vi "SCM1 Ramp and Soak.vi"(2 "Point #":i32, 4 "Parameters":dbl[](array[numeric]) format="%.3e", 5 "GPIB":refnum<visa-resource-name>) -> (0 "Stop":bool, 1 "Data Out":dbl[](array[numeric]) format="%.2f")   [LabVIEW 2025]
doc: "Author: Scott Hannahs <sth@magnet.fsu.edu>\n\nThis software is licensed for use under the “MIT License\"\nCopyright (c) 2025 Scott Hannahs, sth@sth@magnet.sthnet.net\n\nPermission is hereby granted, free of charge, to any person obtaining a copy of this software and associated documentation files (the \"Software\"), to deal in the Software without restriction, including without limitation the rights to use, copy, modify, merge, publish, distribute, sublicense, and/or sell copies of the Software, and to permit persons to whom the Software is furnished to do so, subject to the following conditions: The above copyright notice and this permission notice shall be included in all copies or substantial portions of the Software.\n\nTHE SOFTWARE IS PROVIDED \"AS IS\", WITHOUT WARRANTY OF ANY KIND, EXPRESS OR IMPLIED, INCLUDING BUT NOT LIMITED TO THE WARRANTIES OF MERCHANTABILITY, FITNESS FOR A PARTICULAR PURPOSE AND NONINFRINGEMENT. IN NO EVENT SHALL THE AUTHORS OR COPYRIGHT HOLDERS BE LIABLE FOR ANY CLAIM, DAMAGES OR OTHER LIABILITY, WHETHER IN AN ACTION OF CONTRACT, TORT OR OTHERWISE, ARISING FROM, OUT OF OR IN CONNECTION WITH THE SOFTWARE OR THE USE OR OTHER DEALINGS IN THE SOFTWARE."
panel:
  out "Starting Field":dbl format="%.2f"
  # "Step Size"
  # "Final Field T"
  # "Ramp Rate A/s"
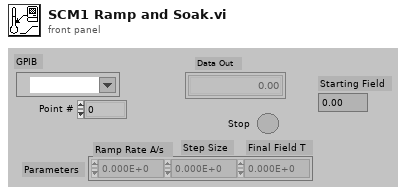
[diagram p1: front panel]
types:
  T1 = cluster{"Parameters[0]":dbl, "Parameters[1]":dbl, "Parameters[2]":dbl}
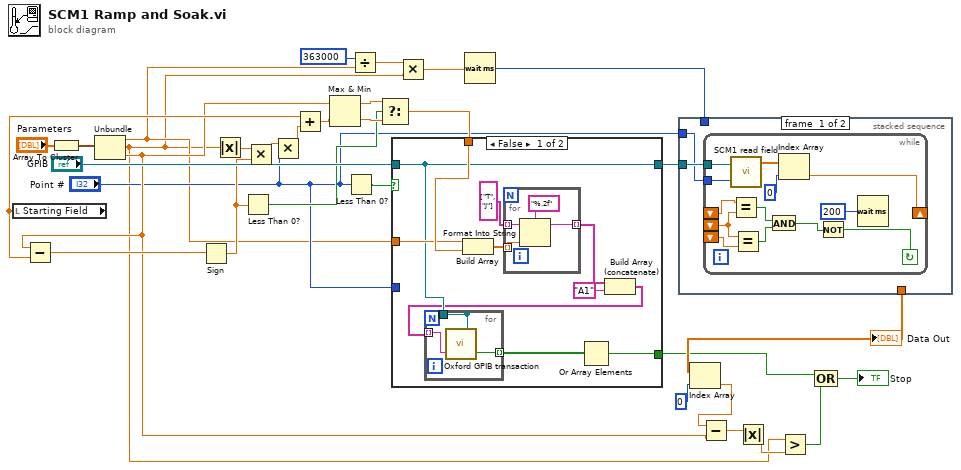
[diagram p0: block diagram]
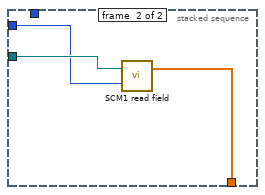
[diagram p2: hidden frame]
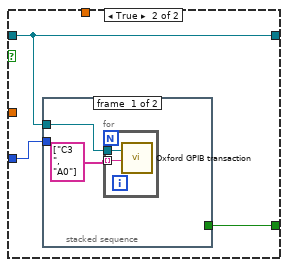
[diagram p3: hidden frame]
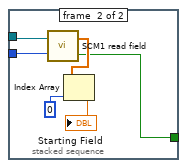
[diagram p4: hidden frame]
diagram:
  n1 = local read "Starting Field"() -> (w21:dbl)
  n2 = Array To Cluster(array="Parameters") -> (cluster=w19:T1)
  n3 = Unbundle(w19) -> ("Parameters[0]"=w6:dbl, "Parameters[1]"=w3:dbl, "Parameters[2]"=w12:dbl)
  n4 = Subtract(x=w12, y=w21) -> (x-y=w30:dbl)
  n5 = Sign(1:w30) -> (0:w23:dbl)
  n6 = Absolute Value(x=w3) -> (abs(x)=w28:dbl)
  n7 = Less Than 0?(x=w23) -> (x < 0?=w22:bool)
  n8 = Multiply(x=w28, y=w23) -> (x*y=w29:dbl)
  n9 = Multiply(x=w29, y="Point #") -> (x*y=w32:dbl)
  n10 = Add(x=w21, y=w32) -> (x+y=w27:dbl)
  n11 = Max & Min(x=w12, y=w27) -> (max(x,y)=w25:dbl, min(x,y)=w24:dbl)
  n12 = Less Than 0?(x="Point #") -> (x < 0?=w20:bool)
  n13 = Divide(x=363000, y=w6) -> (x/y=w4:dbl)
  n14 = Select(t=w25, s=w22, f=w24) -> (s? t:f=w26:dbl)
  n15 = case shown="False" w20 {
    tunnel: "GPIB" -> [w38 w52]
    tunnel: [w38 w52] -> w16
    tunnel: w26 -> [w40 _]
    tunnel: "Point #" -> [_ w51]
    tunnel: [w36 w50] -> w10
    tunnel: w6 -> [w39 _]
    frame False {
      n16 = Build Array(w39, w40) -> (w41:dbl[])
      n17 = for {
        tunnel: w41 -> [w47] mode=indexing
        tunnel: string[] ["T", "J"] -> [w46] mode=indexing
        tunnel: [w49] -> w35 mode=indexing
        n18 = Format Into String(format string="%.2f", initial string=w46, w47) -> (resulting string=w49:string)  [unwired: 1 in, 1 out]
      }
      n19 = Build Array (concatenate)(w35, "A1") -> (w33:string[])
      n20 = for {
        tunnel: [w44] -> _ mode=indexing
        tunnel: w33 -> [w45] mode=indexing
        tunnel: w38 -> [w44]
        tunnel: [w43] -> w37 mode=indexing
        n21 = call "Oxford GPIB transaction.vi"("Command String"=w45, "GPIB Address"=w44) -> ("Stop"=w43:bool)  [unwired: 1 out]
      }
      n22 = Or Array Elements(Boolean array=w37) -> (logical OR=w36:bool)
    }
    frame True {
      n23 = stacked-sequence {
        tunnel: w52 -> [w53 w62]
        tunnel: w51 -> [_ w61]
        tunnel: [_ w57] -> w50
        frame #0 {
          n24 = for {
            tunnel: string[] ["C3 ", "A0"] -> [w56] mode=indexing
            tunnel: w53 -> [w55]
            n25 = call "Oxford GPIB transaction.vi"("Command String"=w56, "GPIB Address"=w55) -> ()  [unwired: 2 out]
          }
        }
        frame #1 {
          n26 = call "SCM1 read field.vi"("Point #"=w61, "Instrument Address"=w62) -> ("Stop"=w57:bool, "Output"=w59:dbl[])
          n27 = Index Array(array=w59, index=0) -> (element=→"Starting Field":dbl)
        }
      }
    }
  }
  n28 = Multiply(x=w4, y=w3) -> (x*y=w2:dbl)
  n29 = Wait (ms)(milliseconds to wait=w2) -> (millisecond timer value=w1:u32)
  n30 = stacked-sequence {
    tunnel: w16 -> [w64 w80]
    tunnel: [_ w79] -> w14
    tunnel: "Point #" -> [w63 w78]
    tunnel: w1 -> [_ _]
    frame #0 {
      n31 = while {
        tunnel: w63 -> [w66]
        shift-left: _ -> [w72]
        shift-left: _ -> [w73]
        shift-left: _ -> [w74]
        shift-right: [w65] -> _
        tunnel: w64 -> [w75]
        stop <- w68 continue-if-true
        n32 = call "SCM1 read field.vi"("Point #"=w66, "Instrument Address"=w75) -> ("Output"=w76:dbl[])  [unwired: 1 out]
        n33 = Equal?(x=w74, y=w73) -> (x = y?=w71:bool)
        n34 = Equal?(x=w73, y=w72) -> (x = y?=w70:bool)
        n35 = And(x=w71, y=w70) -> (x .and. y?=w69:bool)
        n36 = Index Array(array=w76, index=0) -> (element=w65:dbl)
        n37 = Not(x=w69) -> (.not. x?=w68:bool)
        n38 = Wait (ms)(milliseconds to wait=200) -> ()  [unwired: 1 out]
      }
    }
    frame #1 {
      n39 = call "SCM1 read field.vi"("Point #"=w78, "Instrument Address"=w80) -> ("Output"=w79:dbl[])  [unwired: 1 out]
    }
  }
  "Data Out" <- w14
  n40 = Index Array(array=w14, index=0) -> (element=w13:dbl)
  n41 = Subtract(x=w13, y=w12) -> (x-y=w11:dbl)
  n42 = Absolute Value(x=w11) -> (abs(x)=w8:dbl)
  n43 = Greater?(x=w3, y=w8) -> (0:w9:bool)
  n44 = Compound Arithmetic op=OR(w10, w9) -> (→"Stop":bool)
